vi "get_buoy_coords.vi"(8 "error in (no error)":errorcluster, 11 "Enter_Gap in":refnum<class "Enter_Gap.lvclass">) -> (0 "error out":errorcluster, 1 "Buoy 2 Coords":cluster{"X":dbl, "Y":dbl}, 2 "Buoy 1 Coords":cluster{"X":dbl, "Y":dbl}, 3 "Enter_Gap out":refnum<class "Enter_Gap.lvclass">)   [LabVIEW 2011, in "Enter_Gap.lvclass"]
uses:
  Enter_Gap.lvclass
  Enter_Gap.lvclass/Enter_Gap.ctl
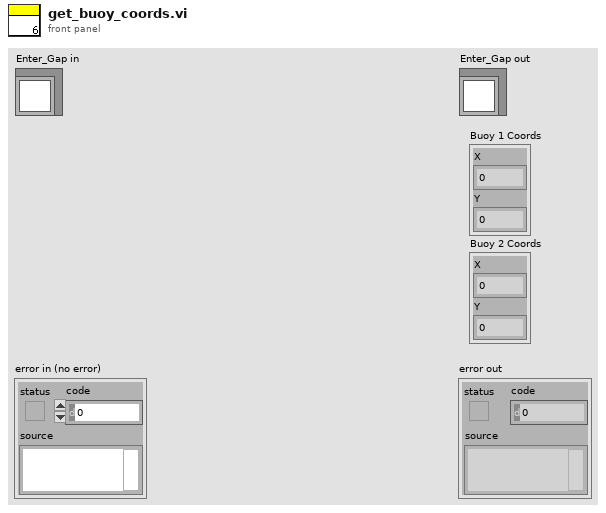
[diagram p1: front panel]
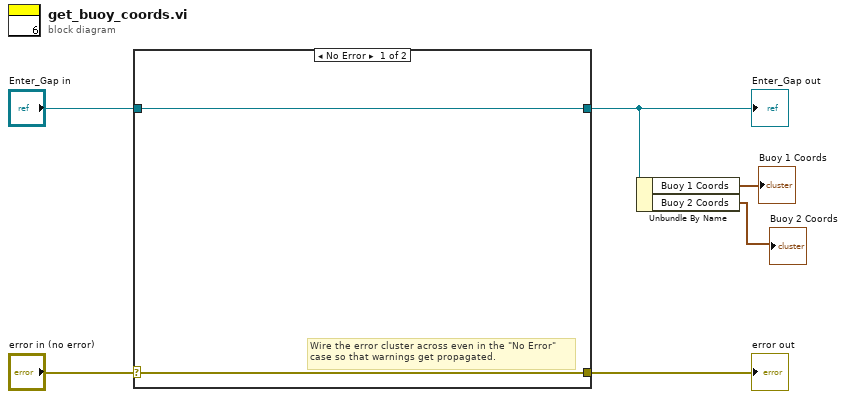
[diagram p0: block diagram]
diagram:
  n1 = case shown="No Error" "error in (no error)" {
    selector: "error in (no error)" -> [w7 w10]
    tunnel: [w7 w10] -> w5
    tunnel: [w8 w9] -> w3
    tunnel: "Enter_Gap in" -> [w8 w9]
    frame No Error {
      # "Wire the error cluster across even in the \"No Error\"\ncase so that warnings get propagated."
    }
    frame Error {
    }
  }
  "error out" <- w5
  "Enter_Gap out" <- w3
  n2 = Unbundle By Name(w3) -> ("Buoy 1 Coords"=→"Buoy 1 Coords":cluster{"X":dbl, "Y":dbl}, "Buoy 2 Coords"=→"Buoy 2 Coords":cluster{"X":dbl, "Y":dbl})
